vi "ScanEngine_SLM.vi"(7 "Action":T2, 8 "Metric Control":T3, 11 "Holo Array In":T1[](array[typedef]) {"Modes"."Amplititute" step=0.05}) -> (0 "Metric Image":sgl[][](array[numeric]), 2 "Metric Result":dbl)   [LabVIEW 2014]
uses:
  Controls/MetricControl_SLM.ctl
  Controls/Scan Metric_SLM.ctl
  Controls/ScanEngineState_SLM.ctl
  Controls/Holo Settings.ctl
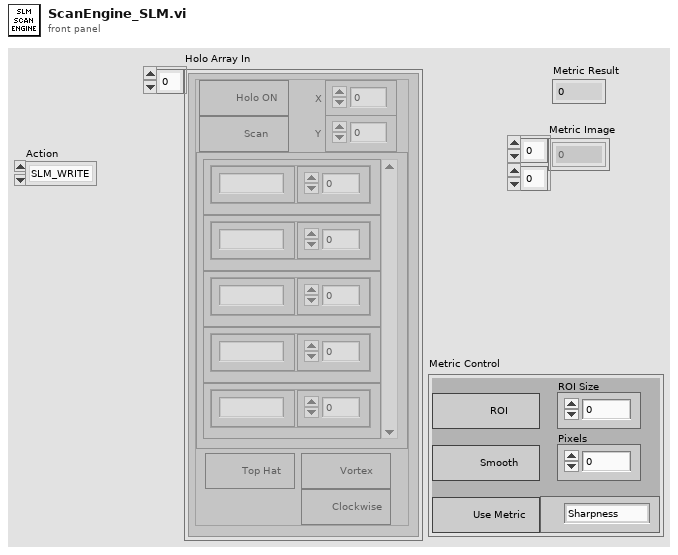
[diagram p1: front panel]
types:
  T1 = typedef "Holo Settings.ctl" = cluster{"Top Hat":bool, "Modes":cluster{"Mode ID":string, "Amplititute":dbl}[], "Vortex":bool, "Clockwise":bool, "X":dbl, "Y":dbl, "Holo ON":bool, "Scan":bool}
  T2 = typedef "ScanEngineState_SLM.ctl" = enum16{"SLM_WRITE", "IMAGE", ""}
  T3 = typedef "MetricControl_SLM.ctl" = cluster{"Use Metric":bool, "SLM Metric":T4, "Smooth":bool, "Pixels":dbl, "ROI":bool, "ROI Size":dbl}
  T4 = typedef "Scan Metric_SLM.ctl" = enum16{"Sharpness", "Brightness", "Combined"}
  T5 = typedef "SLM General Settings.ctl" = cluster{"Holo size (pixels)":i32, "Top hat radius":dbl, "Number of modes":i32, "Bkg gradient X":dbl, "Bkg gradient Y":dbl, "Flat":bool, "Mode Matrix":u16}
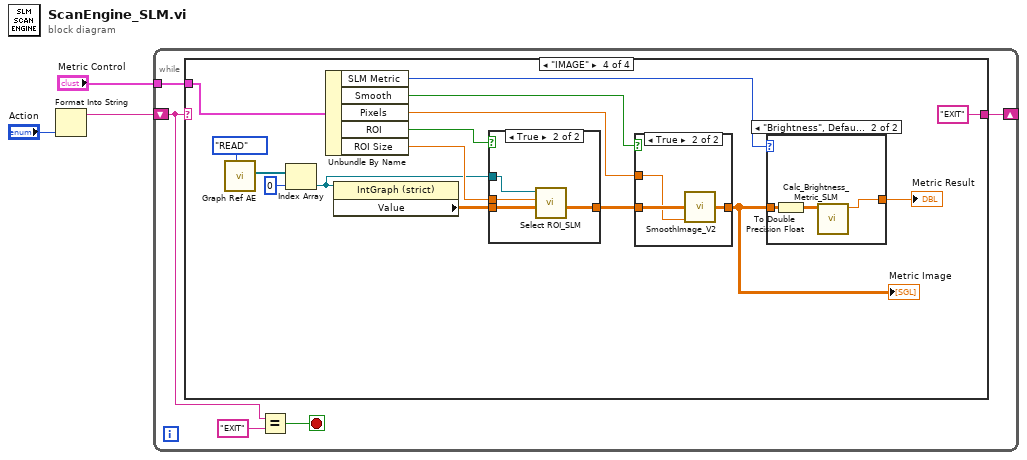
[diagram p0: block diagram]
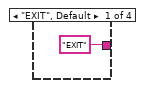
[diagram p2: hidden frame]
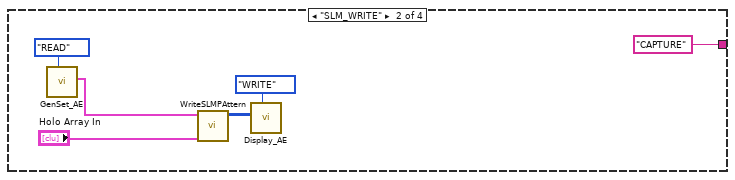
[diagram p3: hidden frame]
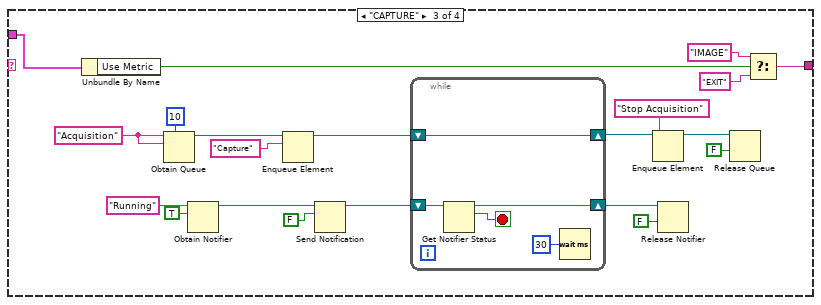
[diagram p4: hidden frame]
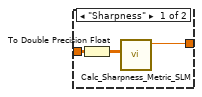
[diagram p6: hidden frame]
diagram:
  n1 = Format Into String("Action") -> (resulting string=w1:string)  [unwired: 3 in, 1 out]
  n2 = while {
    shift-right: [w8] -> _
    shift-left: w1 -> [w7]
    tunnel: "Metric Control" -> [w4]
    stop <- w5 stop-if-true
    n3 = case shown="\"IMAGE\"" w7 {
      tunnel: ["EXIT" "CAPTURE" w33 "EXIT"] -> w8
      tunnel: w4 -> [_ _ w22 w53]
      frame "EXIT", Default {
      }
      frame "SLM_WRITE" {
        n4 = call "GenSet_AE.vi"("Enum"=enum16{"READ", "WRITE"}."READ") -> ("General settings Out"=w12:T5)  [unwired: 10 in]
        n5 = call "WriteSLMPAttern.vi"("Holo Array"="Holo Array In", "General settings"=w12) -> ("Display Array"=w11:u8[][])  [unwired: 9 in]
        n6 = call "Display_AE.vi"("Action"=enum16{"READ", "WRITE"}."WRITE", "Display Array In"=w11) -> ()  [unwired: 9 in, 1 out]
      }
      frame "CAPTURE" {
        w30 = "Acquisition" ("name (unnamed)")
        n7 = Unbundle By Name(w22) -> ("Use Metric"=w21:bool)
        n8 = Obtain Queue(max queue size (-1, unlimited)=10, name (unnamed)=w30, element data type=w30) -> (queue out=w28:refnum<queue>)  [unwired: 2 in, 2 out]
        n9 = Obtain Notifier(name (unnamed)="Running", notification data type=TRUE) -> (notifier out=w25:refnum<notifier>)  [unwired: 2 in, 2 out]
        n10 = Enqueue Element(queue=w28, element="Capture") -> (queue out=w18:refnum<queue>)  [unwired: 2 in, 2 out]
        n11 = Send Notification(notification=FALSE, notifier=w25) -> (notifier out=w34:refnum<notifier>)  [unwired: 1 in, 1 out]
        n12 = while {
          shift-right: [w37] -> w19
          shift-left: w18 -> [w37]
          shift-right: [w38] -> w24
          shift-left: w34 -> [w41]
          stop <- w40 stop-if-true
          n13 = Get Notifier Status(notifier=w41) -> (notifier out=w38:refnum<notifier>, current notification=w40:bool)  [unwired: 1 in, 3 out]
          n14 = Wait (ms)(milliseconds to wait=u32 30) -> ()  [unwired: 1 out]
        }
        n15 = Enqueue Element(queue=w19, element="Stop Acquisition") -> (queue out=w17:refnum<queue>)  [unwired: 2 in, 2 out]
        n16 = Release Notifier(notifier=w24, force destroy? (F)=FALSE) -> ()  [unwired: 1 in, 3 out]
        n17 = Release Queue(queue=w17, force destroy? (F)=FALSE) -> ()  [unwired: 1 in, 3 out]
        n18 = Select(t="IMAGE", s=w21, f="EXIT") -> (s? t:f=w33:string)
      }
      frame "IMAGE" {
        n19 = call "Graph Ref AE.vi"("Action"=enum16{"READ", "WRITE"}."READ") -> ("Graph Ref Out"=w48:refnum<vi>[])  [unwired: 10 in]
        n20 = Index Array(array=w48, index=0) -> (element=w42:refnum<vi>)
        n21 = Unbundle By Name(w53) -> ("SLM Metric"=w52:T4, "Smooth"=w50:bool, "Pixels"=w51:dbl, "ROI"=w46:bool, "ROI Size"=w43:dbl)
        n22 = property class="IntGraph (strict)"(reference=w42) -> ("Value"=w44:sgl[][])  [unwired: 1 in, 2 out]
        n23 = case shown="True" w46 {
          tunnel: w44 -> [w57 w61]
          tunnel: [w57 w60] -> w45
          tunnel: w43 -> [_ w59]
          tunnel: w42 -> [_ w58]
          frame False {
          }
          frame True {
            n24 = call "Select ROI_SLM.vi"("Array In"=w61, "ROI Size"=w59, "IntensityGraph in"=w58) -> ("ROI"=w60:sgl[][])  [unwired: 8 in]
          }
        }
        n25 = case shown="True" w50 {
          tunnel: w45 -> [w68 w71]
          tunnel: [w68 w70] -> w56
          tunnel: w51 -> [_ w69]
          frame False {
          }
          frame True {
            n26 = call "SmoothImage_V2.vi"("Image IN"=w71, "Sigma (Radius)"=w69) -> ("Smoothed Image"=w70:sgl[][])  [unwired: 13 in]
          }
        }
        "Metric Image" <- w56
        n27 = case shown="\"Brightness\", Default" w52 {
          tunnel: w56 -> [w64 w67]
          tunnel: [w62 w66] -> w54
          frame "Sharpness" {
            n28 = To Double Precision Float(number=w64) -> (double precision float=w63:dbl[][])
            n29 = call "Calc_Sharpness_Metric_SLM.vi"("AC Image"=w63) -> ("Numeric out"=w62:dbl)  [unwired: 10 in]
          }
          frame "Brightness", Default {
            n30 = To Double Precision Float(number=w67) -> (double precision float=w65:dbl[][])
            n31 = call "Calc_Brightness_Metric_SLM.vi"("Image In"=w65) -> ("Brightness"=w66:dbl)  [unwired: 10 in]
          }
        }
        "Metric Result" <- w54
      }
    }
    n32 = Equal?(x=w7, y="EXIT") -> (x = y?=w5:bool)
  }
